vi "MHEX_CUIT_CRC_CHECK.vi"(8 "Error In":errorcluster, 11 "string in":string) -> (0 "Error Out":errorcluster)   [LabVIEW 2018]
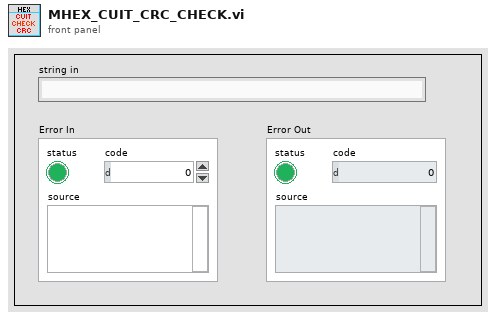
[diagram p1: front panel]
types:
  T1 = typedef "MLLC_Error.ctl" = errorcluster
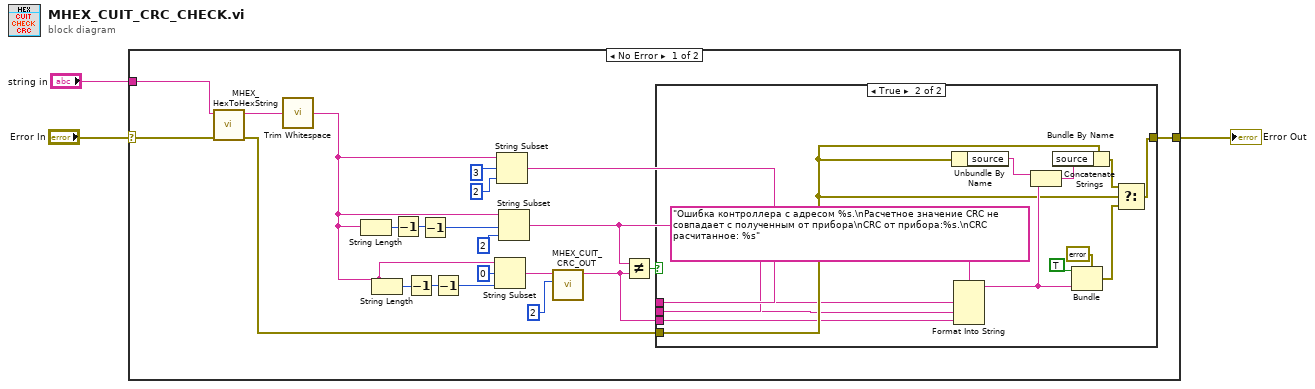
[diagram p0: block diagram]
diagram:
  n1 = case shown="No Error" "Error In" {
    selector: "Error In" -> [w11 w40]
    tunnel: "string in" -> [w5 _]
    tunnel: [w13 w40] -> w2
    frame No Error {
      n2 = call "MHEX_HexToHexString.vi"("error in (no error)"=w11, "STRING HEX"=w5) -> ("error out"=w17:T1, "String out"=w4:string)  [unwired: 7 in, 1 out]
      n3 = call <vilib>:"Trim Whitespace.vi"("string"=w4) -> ("trimmed string"=w8:string)  [unwired: 1 in]
      n4 = String Length(string=w8) -> (length=w19:i32)
      n5 = String Length(string=w8) -> (length=w21:i32)
      n6 = Decrement(x=w19) -> (x-1=w18:i32)
      n7 = Decrement(x=w21) -> (x-1=w20:i32)
      n8 = Decrement(x=w18) -> (x-1=w22:i32)
      n9 = Decrement(x=w20) -> (x-1=w24:i32)
      n10 = String Subset(string=w8, offset (0)=0 ("length (rest)"), length (rest)=w24) -> (substring=w10:string)
      n11 = String Subset(string=w8, offset (0)=3, length (rest)=2 ("length (rest)")) -> (substring=w14:string)
      n12 = String Subset(string=w8, offset (0)=w22, length (rest)=2 ("offset (0)")) -> (substring=w12:string)
      n13 = call "MHEX_CUIT_CRC_OUT.vi"("width (-)"=i16 2, "String"=w10) -> ("hex integer string"=w9:string)  [unwired: 8 in, 1 out]
      n14 = Not Equal?(x=w12, y=w9) -> (x != y?=w7:bool)
      n15 = case shown="True" w7 {
        tunnel: [w26 w31] -> w13
        tunnel: w9 -> [_ w27]
        tunnel: w12 -> [_ w28]
        tunnel: w17 -> [w26 w30]
        tunnel: w14 -> [_ w29]
        frame False {
        }
        frame True {
          n16 = Unbundle By Name(w30) -> ("source"=w36:string)
          n17 = Format Into String(format string="Ошибка контроллера с адресом %s.\nРасчетное значение CRC не совпадает с полученным от прибора\nCRC от прибора:%s.\nCRC  расчитанное: %s", w29, w28, w27) -> (resulting string=w34:string)  [unwired: 2 in, 1 out]
          n18 = Concatenate Strings(w36, w34) -> (w35:string)
          n19 = Bundle By Name(cluster=w30, "source"=w35) -> (w33:T1)
          n20 = Bundle(cluster=errorcluster {"status"=FALSE, "code"=0, "source"=""} ("error out"), "status"=TRUE ("Status"), "source"=w34) -> (w32:errorcluster)  [unwired: 1 in]
          n21 = Select(t=w33, s=w30, f=w32) -> (s? t:f=w31:T1)
        }
      }
    }
    frame Error {
    }
  }
  "Error Out" <- w2
